vi "test - seperated but same session.vi"(8 "error in (no error)":errorcluster, 11 "TestCase in":refnum<class "labview-config-library.lvclass">) -> (0 "error out":errorcluster, 3 "TestCase out":refnum<class "labview-config-library.lvclass">)   [LabVIEW 2017, in "labview-config-library.lvclass"]
uses:
  labview-config-library.lvclass
  <vilib>/addons/_JKI Toolkits/VI Tester/TestCase.llb/TestCase.lvclass
  INI-Static-Variable-Support/LabVIEW-Config/LabVIEW-Config.lvclass
  C:/Program Files (x86)/National Instruments/LabVIEW 2017/vi.lib/addons/_JKI Toolkits/VI Tester/TestCase.llb/TestCase.lvclass
panel:
  in  "Tab Control":enum32{"Page 1", "Page 2", "Page 3"}(tab)
  out "Section Names":string[](array[string])
  out "Key Names":string[](array[string])
  out "Array":string[](array[string])
  out "Key Names 2":string[](array[string])
  out "Array 2":string[](array[string])
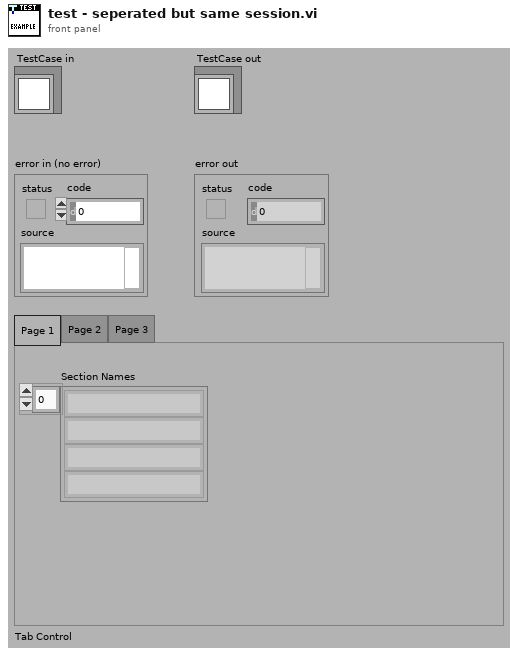
[diagram p1: front panel]
types:
  T1 = typedef "LabVIEW-Config.lvlib/LabVIEW-Config.lvclass/Config.ctl" = cluster{"Path":path, "Lines":string[], "Tokens":T2[], "Modified?":bool, "Cache":cluster{"Valid?":bool, "Key Information":T3[]}}
  T2 = typedef "LabVIEW-Config.lvlib/LabVIEW-Config.lvclass/LineToken.ctl" = enum8{"comment", "section", "key", "more"}
  T3 = typedef "LabVIEW-Config.lvlib/LabVIEW-Config.lvclass/KeyInfo.ctl" = cluster{"Key Indexes":cluster{"Indexes":i32[]}[], "Session Found?":bool, "Key found?":bool, "Session Index":i32}
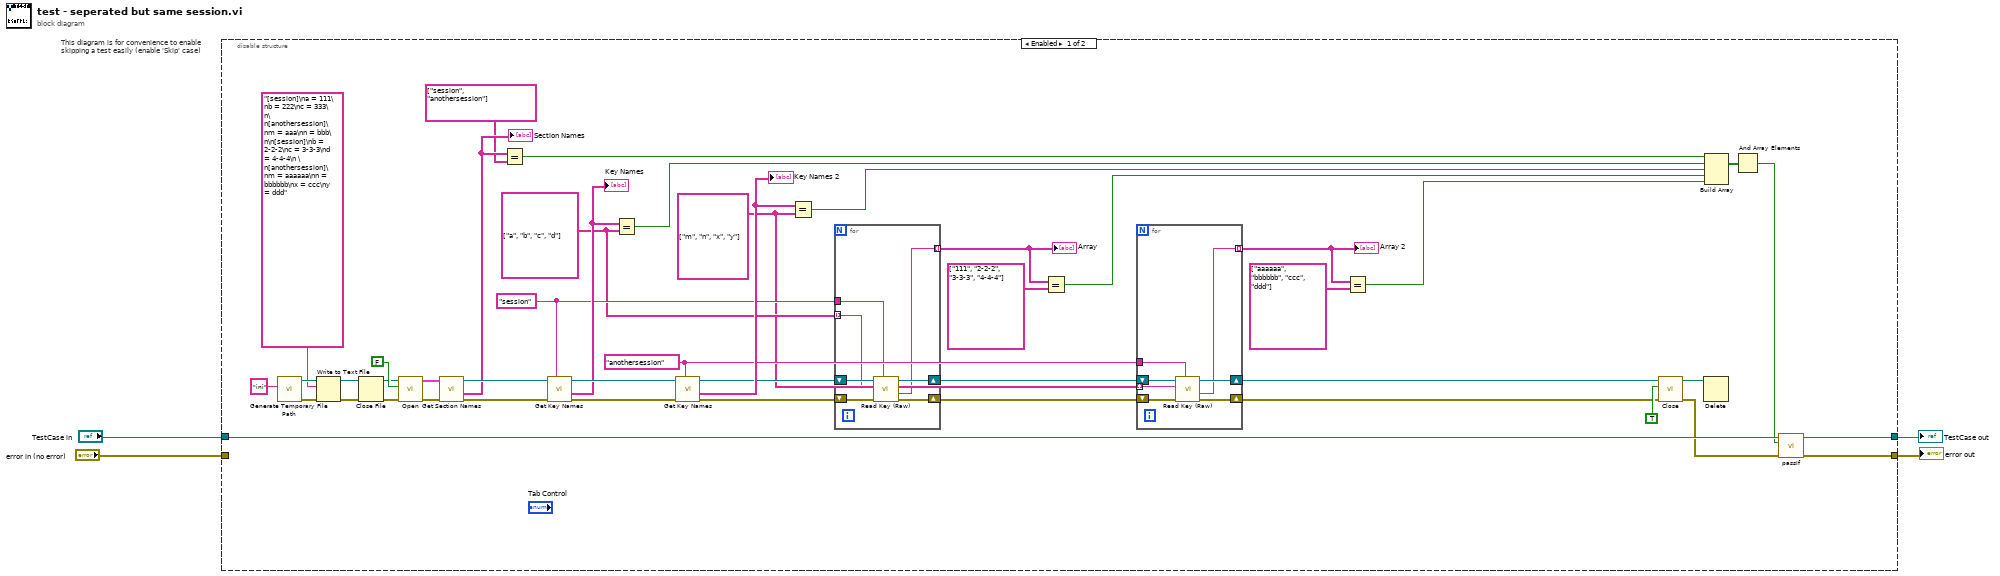
[diagram p0: block diagram]
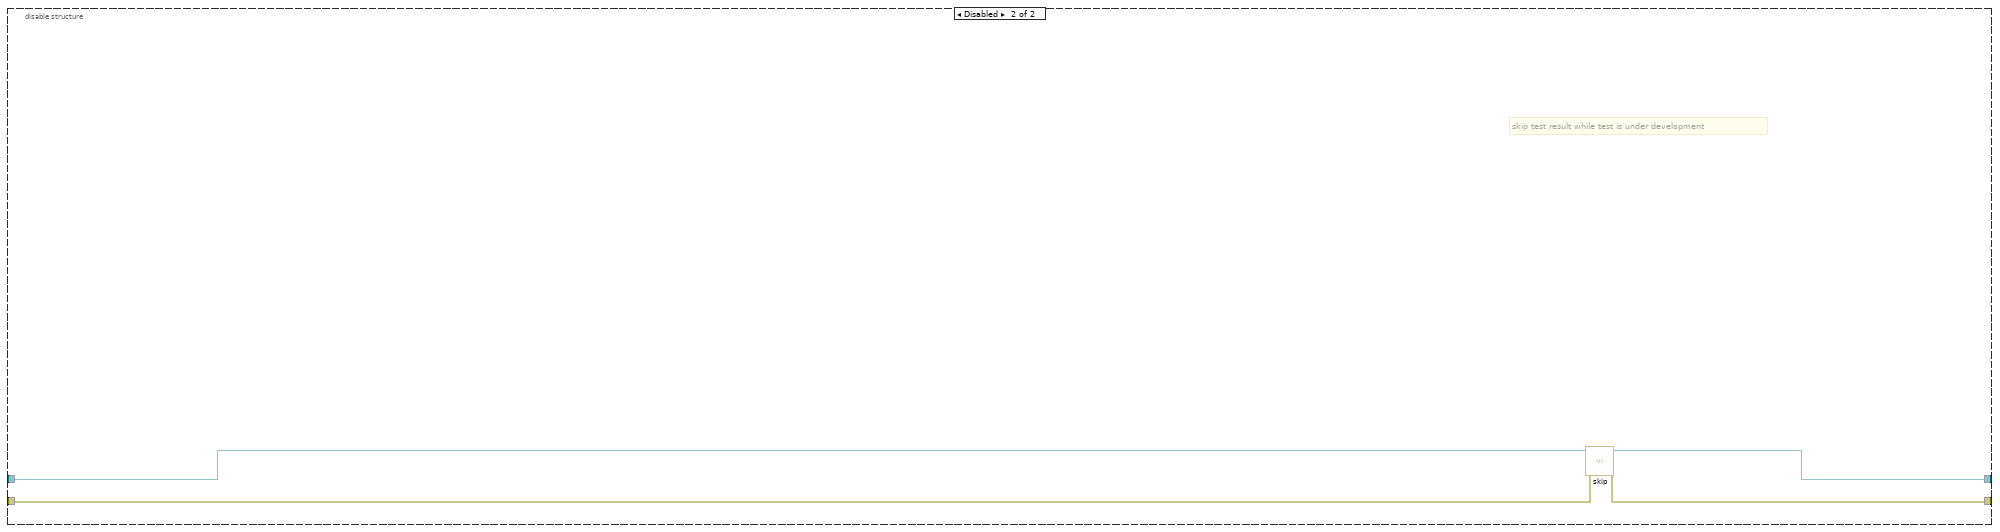
[diagram p2: hidden frame]
diagram:
  n1 = disable-structure "This diagram is for convenience to enable skipping a test easily (enable 'Skip' case)" shown="Enabled" {
    disable-tunnel: "TestCase in" -> [w50 w68]
    disable-tunnel: [w49 w66] -> w1
    disable-tunnel: [w48 w67] -> w3
    disable-tunnel: "error in (no error)" -> [_ w65]
    frame Enabled {
      w8 = string[] ["m", "n", "x", "y"] ("Key Names 2")
      w17 = string[] ["a", "b", "c", "d"] ("Key Names")
      w9 = "anothersession" ("Section Name")
      w18 = "session" ("Section Name")
      # "Create temporary ini file"
      n2 = call <vilib>:"Generate Temporary File Path.vi"("Temporary File Extension (tmp)"="ini") -> ("error out"=w45:errorcluster, "Unique Temporary File Path"=w42:path)  [unwired: 9 in]
      n3 = Write to Text File(file (use dialog)=w42, text="[session]\na = 111\nb = 222\nc = 333\n\n[anothersession]\nm = aaa\nn = bbb\n\n[session]\nb = 2-2-2\nc = 3-3-3\nd = 4-4-4\n \n[anothersession]\nm = aaaaaa\nn = bbbbbb\nx = ccc\ny = ddd", error in=w45) -> (refnum out=w41:refnum<file>, error out=w43:errorcluster)  [unwired: 1 in, 1 out]
      n4 = Close File(refnum=w41, error in=w43) -> (path=w37:path, error out=w38:errorcluster)
      n5 = call "Open.vi"("error in (no error)"=w38, "Create if not exists? (T)"=FALSE, "Path"=w37) -> ("error out"=w34:errorcluster, "Config"=w35:T1)  [unwired: 5 in, 2 out]
      n6 = call "Get Section Names.vi"("error in (no error)"=w34, "Config in"=w35) -> ("error out"=w30:errorcluster, "Section Names"=w29:string[], "Config out"=w31:refnum<class "LabVIEW-Config.lvclass">)  [unwired: 7 in]
      "Section Names" <- w29
      n7 = Equal?(x=w29, y=string[] ["session", "anothersession"]) -> (x = y?=w27:bool)
      n8 = call "Get Key Names.vi"("Section Name"=w18, "error in (no error)"=w30, "Config in"=w31) -> ("error out"=w33:errorcluster, "Key Names"=w25:string[], "Config out"=w32:refnum<class "LabVIEW-Config.lvclass">)  [unwired: 5 in, 1 out]
      "Key Names" <- w25
      n9 = Equal?(x=w25, y=w17) -> (x = y?=w24:bool)
      n10 = call "Get Key Names.vi"("Section Name"=w9, "error in (no error)"=w33, "Config in"=w32) -> ("error out"=w19:errorcluster, "Key Names"=w23:string[], "Config out"=w20:refnum<class "LabVIEW-Config.lvclass">)  [unwired: 5 in, 1 out]
      "Key Names 2" <- w23
      n11 = Equal?(x=w23, y=w8) -> (x = y?=w22:bool)
      n12 = for {
        tunnel: w18 -> [w53]
        shift-right: [w54] -> w11
        shift-left: w20 -> [w57]
        shift-right: [w55] -> w10
        shift-left: w19 -> [w56]
        tunnel: w17 -> [w52] mode=indexing
        tunnel: [w51] -> w15 mode=indexing
        n13 = call "Read Key (Raw).vi"("Section Name"=w53, "error in (no error)"=w56, "Key Name"=w52, "Config in"=w57) -> ("error out"=w55:errorcluster, "Content"=w51:string, "Config out"=w54:refnum<class "LabVIEW-Config.lvclass">)  [unwired: 4 in, 1 out]
      }
      "Array" <- w15
      n14 = Equal?(x=w15, y=string[] ["111", "2-2-2", "3-3-3", "4-4-4"] ("Key Names")) -> (x = y?=w14:bool)
      n15 = for {
        tunnel: w9 -> [w60]
        shift-right: [w61] -> w6
        shift-left: w11 -> [w64]
        shift-right: [w62] -> w5
        shift-left: w10 -> [w63]
        tunnel: w8 -> [w59] mode=indexing
        tunnel: [w58] -> w13 mode=indexing
        n16 = call "Read Key (Raw).vi"("Section Name"=w60, "error in (no error)"=w63, "Key Name"=w59, "Config in"=w64) -> ("error out"=w62:errorcluster, "Content"=w58:string, "Config out"=w61:refnum<class "LabVIEW-Config.lvclass">)  [unwired: 4 in, 1 out]
      }
      "Array 2" <- w13
      n17 = Equal?(x=w13, y=string[] ["aaaaaa", "bbbbbb", "ccc", "ddd"] ("Key Names")) -> (x = y?=w7:bool)
      n18 = call "Close.vi"("error in (no error)"=w5, "Write if modified? (T)"=TRUE, "Config"=w6) -> ("error out"=w36:errorcluster, "Path"=w39:path)  [unwired: 7 in]
      n19 = Delete(path (use dialog)=w39) -> ()  [unwired: 4 in, 3 out]
      n20 = Build Array(w27, w24, w22, w14, w7) -> (w26:bool[])
      n21 = And Array Elements(Boolean array=w26) -> (logical AND=w21:bool)
      n22 = call-dynamic "passIf.vi"("error in (no error)"=w36, "pass"=w21, "TestCase in"=w50) -> ("error out"=w48:errorcluster, "TestCase out"=w49:refnum<class "labview-config-library.lvclass">)  [unwired: 7 in]
    }
    frame Disabled {
      # "skip test result while test is under development"
      n23 = call <vilib>:"skip.vi"("error in (no error)"=w65, "TestCase in"=w68) -> ("error out"=w67:errorcluster, "TestCase out"=w66:refnum<class "labview-config-library.lvclass">)  [unwired: 8 in]
    }
  }
  "error out" <- w3
  "TestCase out" <- w1
